vi "PlanVirtualStave.vi"(7 "Stave Locking Points [mm]":dbl[][](array[numeric])=[[0.0, 0.0, 0.0], [280.05, 0.0, 0.0], [574.05, 0.0, 0.0], [868.05, 0.0, 0.0], [1162.05, 0.0, 0.0]], 8 "Working height [mm]":dbl, 10 "Module fiducial marker":T3(ring), 11 "Tape Type":enum16{"Stereo", "Axial"}(ring)=enum."Axial") -> (0 "Module fiducials in the Stave's basis":T1(graph)=[{"Generated List of Module Coordinates"=[-7.69, 87.79, 87.79, -7.69, 90.31, 185.79000000000002, 185.79000000000002, 90.31, 188.31, 283.79, 283.79, 188.31, 286.31, 381.79, 381.79, 286.31, 384.31, 479.79, 479.79, 384.31, 482.31, 577.79, 577.79, 482.31, 580.31, 675.79, 675.79, 580.31, 678.31, 773.79, 773.79, 678.31, 776.31, 871.79, 871.79, 776.31, 874.31, 969.79, 969.79, 874.31, 972.31, 1067.79, 1067.79, 972.31, 1070.31, 1165.79, 1165.79, 1070.31, 1168.31, 1263.79, 1263.79, 1168.31], "Generated List of Module Coordinates"=[-16.132, -16.132, -113.21200000000002, -113.21200000000002, -16.132, -16.132, -113.21200000000002, -113.21200000000002, -16.132, -16.132, -113.21200000000002, -113.21200000000002, -16.132, -16.132, -113.21200000000002, -113.21200000000002, -16.132, -16.132, -113.21200000000002, -113.21200000000002, -16.132, -16.132, -113.21200000000002, -113.21200000000002, -16.132, -16.132, -113.21200000000002, -113.21200000000002, -16.132, -16.132, -113.21200000000002, -113.21200000000002, -16.132, -16.132, -113.21200000000002, -113.21200000000002, -16.132, -16.132, -113.21200000000002, -113.21200000000002, -16.132, -16.132, -113.21200000000002, -113.21200000000002, -16.132, -16.132, -113.21200000000002, -113.21200000000002, -16.132, -16.132, -113.21200000000002, -113.21200000000002]}, {"Generated List of Module Coordinates"=[0.0, 280.05, 574.05, 868.05, 1162.05], "Generated List of Module Coordinates"=[0.0, 0.0, 0.0, 0.0, 0.0]}], 3 "Generated List: Coordinates of Fiducials on Modules":dbl[][](array[numeric])=[[-7.69, -16.132, 0.0], [87.79, -16.132, 0.0], [87.79, -113.21200000000002, 0.0], [-7.69, -113.21200000000002, 0.0], [90.31, -16.132, 0.0], [185.79000000000002, -16.132, 0.0], [185.79000000000002, -113.21200000000002, 0.0], [90.31, -113.21200000000002, 0.0], [188.31, -16.132, 0.0], [283.79, -16.132, 0.0], [283.79, -113.21200000000002, 0.0], [188.31, -113.21200000000002, 0.0], [286.31, -16.132, 0.0], [381.79, -16.132, 0.0], [381.79, -113.21200000000002, 0.0], [286.31, -113.21200000000002, 0.0], [384.31, -16.132, 0.0], [479.79, -16.132, 0.0], [479.79, -113.21200000000002, 0.0], [384.31, -113.21200000000002, 0.0], [482.31, -16.132, 0.0], [577.79, -16.132, 0.0], [577.79, -113.21200000000002, 0.0], [482.31, -113.21200000000002, 0.0], [580.31, -16.132, 0.0], [675.79, -16.132, 0.0], [675.79, -113.21200000000002, 0.0], [580.31, -113.21200000000002, 0.0], [678.31, -16.132, 0.0], [773.79, -16.132, 0.0], [773.79, -113.21200000000002, 0.0], [678.31, -113.21200000000002, 0.0], [776.31, -16.132, 0.0], [871.79, -16.132, 0.0], [871.79, -113.21200000000002, 0.0], [776.31, -113.21200000000002, 0.0], [874.31, -16.132, 0.0], [969.79, -16.132, 0.0], [969.79, -113.21200000000002, 0.0], [874.31, -113.21200000000002, 0.0], [972.31, -16.132, 0.0], [1067.79, -16.132, 0.0], [1067.79, -113.21200000000002, 0.0], [972.31, -113.21200000000002, 0.0], [1070.31, -16.132, 0.0], [1165.79, -16.132, 0.0], [1165.79, -113.21200000000002, 0.0], [1070.31, -113.21200000000002, 0.0], [1168.31, -16.132, 0.0], [1263.79, -16.132, 0.0], [1263.79, -113.21200000000002, 0.0], [1168.31, -113.21200000000002, 0.0]])   [LabVIEW 2016]
panel:
  out "output cluster":cluster{dbl[], dbl[]}
  out "Y centreline":dbl
  out "Distance to EOS, x [mm]":dbl=-7.69
  in  "Module centre [mm]":T2
  in  "N modules":dbl=13.0
  out "Distance to EOS, y [mm]":dbl=-16.132
  in  "Module width [mm]":dbl=97.54
  in  "Module pitch [mm]":dbl=98.0
  # "Based on Sutcliffe Drawings:\n\nDistance to EOS, axial = [ -7.69, -16.132 ]\nstereo = [ -9.591, 115.081 ]"
  # "Provided by Camera Calibration:"
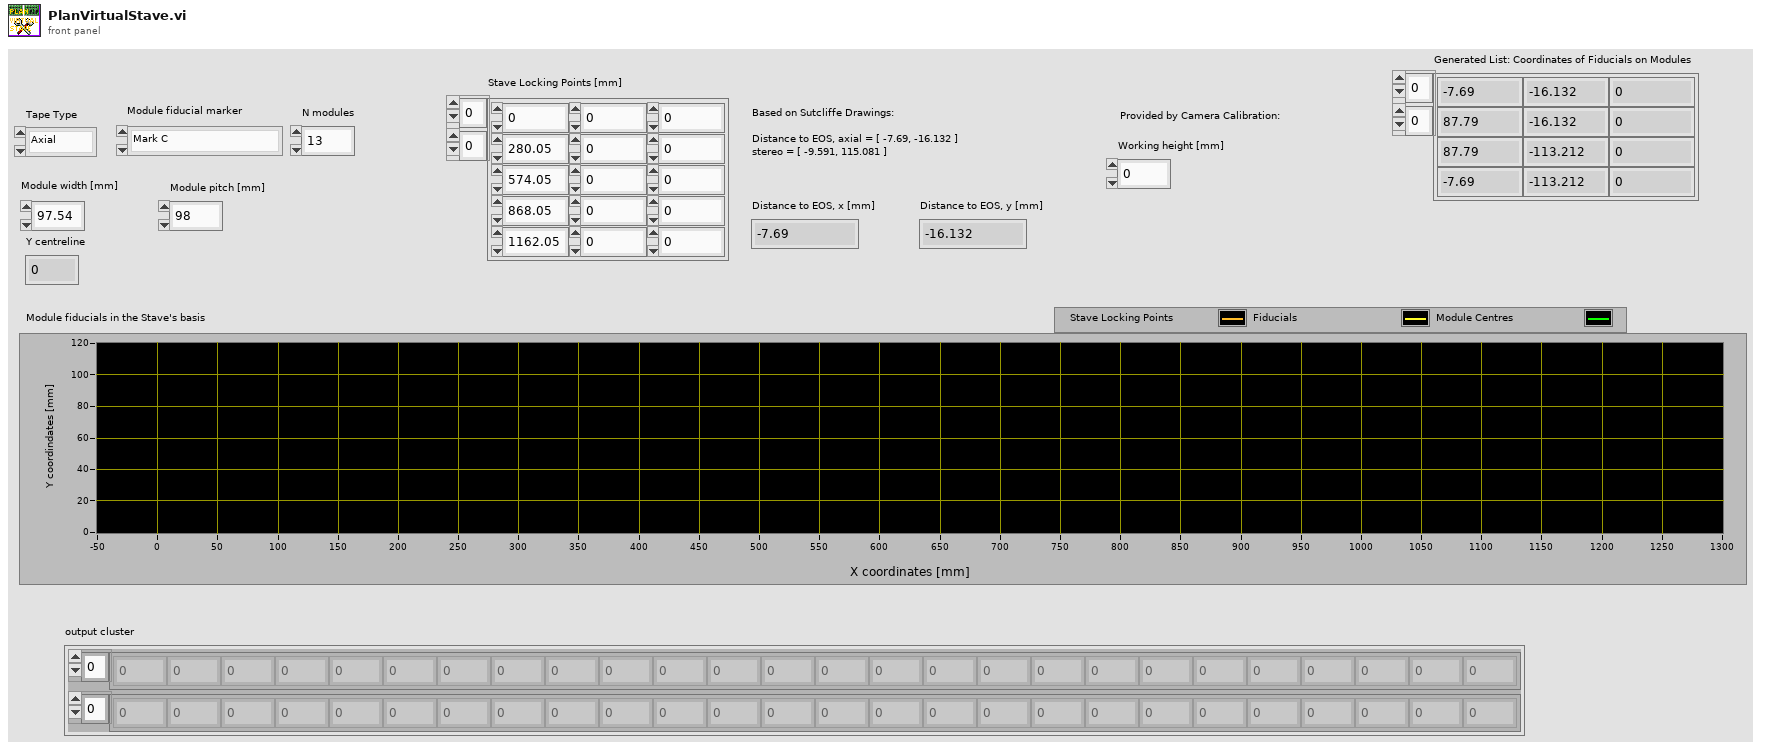
[diagram p1: front panel]
types:
  T1 = cluster{"Generated List of Module Coordinates":dbl[], "Generated List of Module Coordinates":dbl[]}[]
  T2 = cluster{"X [mm]":dbl, "Y [mm]":dbl, "Z [mm]":dbl}
  T3 = enum16{"Mark C", "Mark B", "Strip Corner", "[None]"}
  T4 = cluster{"Generated List of Module Coordinates":dbl[], "Generated List of Module Coordinates":dbl[]}
  T5 = cluster{"Stave Locking Points [mm]":dbl[], "Stave Locking Points [mm]":dbl[]}
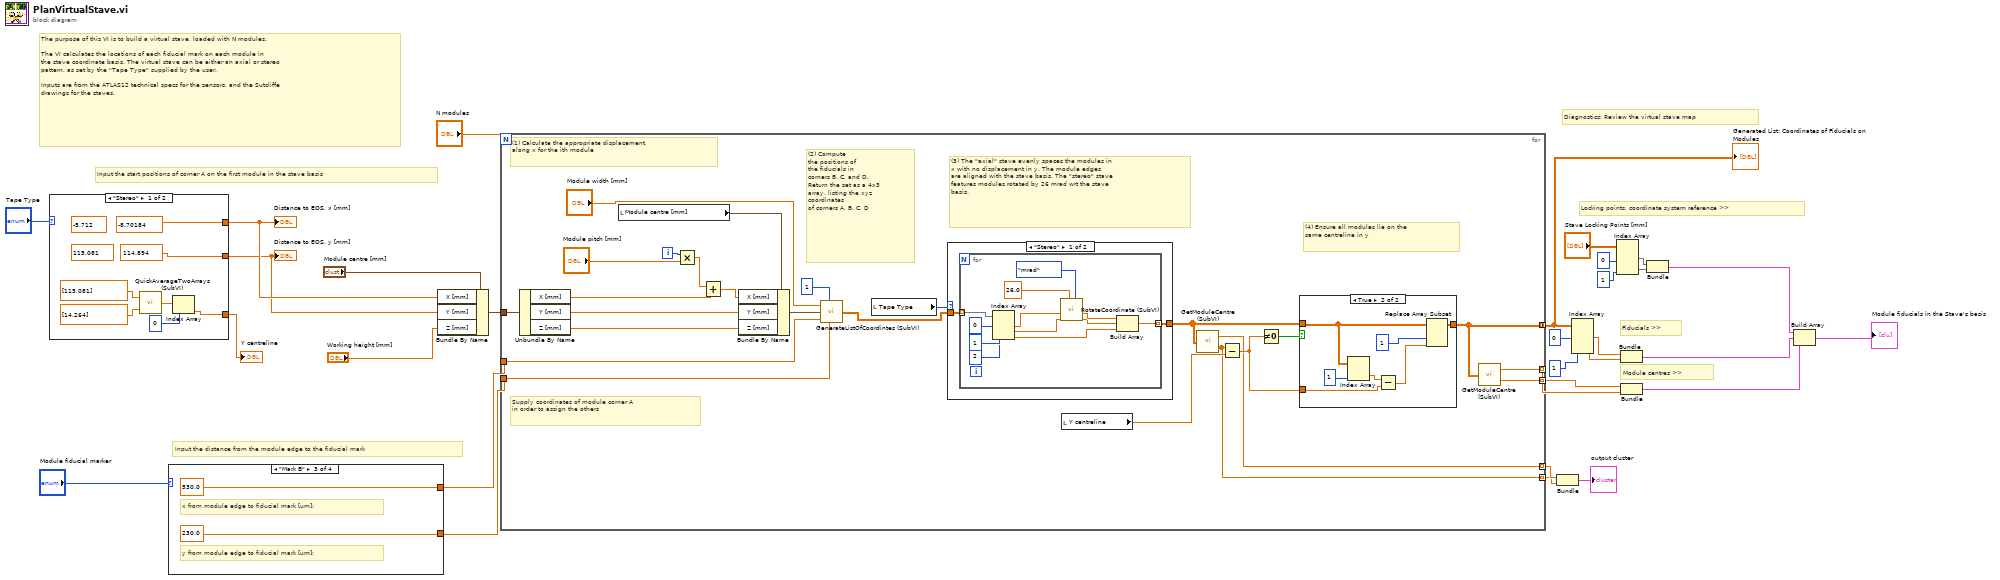
[diagram p0: block diagram]
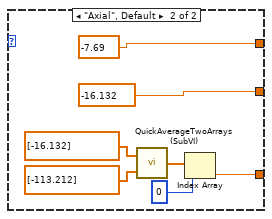
[diagram p2: hidden frame]
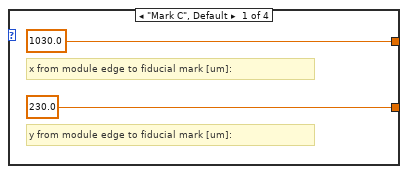
[diagram p5: hidden frame]
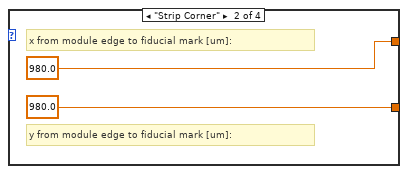
[diagram p6: hidden frame]
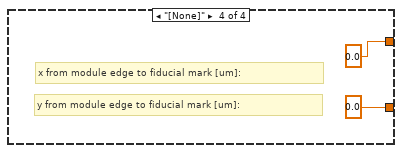
[diagram p7: hidden frame]
diagram:
  # "Locking points, coordinate system reference >>"
  # "Module centres >>"
  # "Fiducials >>"
  # "Diagnostics: Review the virtual stave map"
  # "Input the start positions of corner A on the first module in the stave basis"
  # "Input the distance from the module edge to the fiducial mark"
  # "The purpose of this VI is to build a virtual stave, loaded with N modules.\n\nThe VI calculates the locations of each fiducial mark on each module in \nthe stave coordinate basis. The virtual stave can be either an axial or stereo \npattern, as set by the \"Tape Type\" supplied by the user.\n\nInputs are from the ATLAS12 technical specs for the sensors, and the Sutcliffe\ndrawings for the staves."
  n1 = case shown="\"Stereo\"" "Tape Type" {
    tunnel: [-8.70184 -7.69] -> w15
    tunnel: [114.894 -16.132] -> w14
    tunnel: [w31 w38] -> w4
    frame "Stereo" {
      (unwired) 115.081
      (unwired) -5.712
      n2 = call "QuickAverageTwoArrays (SubVI).vi"("B"=dbl[] [14.264], "A"=dbl[] [115.081]) -> ("Average of A and B"=w33:dbl[])
      n3 = Index Array(array=w33, index=0) -> (element=w31:dbl)
    }
    frame "Axial", Default {
      n4 = call "QuickAverageTwoArrays (SubVI).vi"("B"=dbl[] [-113.212], "A"=dbl[] [-16.132]) -> ("Average of A and B"=w40:dbl[])
      n5 = Index Array(array=w40, index=0) -> (element=w38:dbl)
    }
  }
  "Distance to EOS, y [mm]" <- w14
  "Distance to EOS, x [mm]" <- w15
  "Y centreline" <- w4
  n6 = case shown="\"Mark B\"" "Module fiducial marker" {
    tunnel: [1030.0 980.0 530.0 0.0] -> w29
    tunnel: [230.0 980.0 230.0 0.0] -> w28
    frame "Mark C", Default {
      # "y from module edge to fiducial mark [um]:"
      # "x from module edge to fiducial mark [um]:"
    }
    frame "Strip Corner" {
      # "y from module edge to fiducial mark [um]:"
      # "x from module edge to fiducial mark [um]:"
    }
    frame "Mark B" {
      # "y from module edge to fiducial mark [um]:"
      # "x from module edge to fiducial mark [um]:"
    }
    frame "[None]" {
      # "y from module edge to fiducial mark [um]:"
      # "x from module edge to fiducial mark [um]:"
    }
  }
  n7 = Bundle By Name(cluster="Module centre [mm]", "X [mm]"=w15, "Y [mm]"=w14, "Z [mm]"="Working height [mm]") -> (w22:T2)
  n8 = for {
    N: "N modules" -> [_]
    tunnel: w29 -> [w66]
    tunnel: w28 -> [w76]
    tunnel: w22 -> [w65]
    tunnel: [w58] -> w13 mode=concatenating
    tunnel: [w57] -> w10 mode=indexing
    tunnel: [w56] -> w9 mode=indexing
    tunnel: [w54] -> w3 mode=indexing
    tunnel: [w53] -> w2 mode=indexing
    i -> [w75]
    # "(4) Ensure all modules lie on the \nsame centreline in y"
    # "(3) The \"axial\" stave evenly spaces the modules in \nx with no displacement in y. The module edges \nare aligned with the stave basis. The \"stereo\" stave \nfeatures modules rotated by 26 mrad wrt the stave\nbasis."
    # "(2) Compute\nthe positions of \nthe fiducials in \ncorners B, C, and D. \nReturn the set as a 4x3\narray, listing the xyz \ncoordinates\nof corners A, B, C, D"
    # "(1) Calculate the appropriate displacement \nalong x for the ith module"
    # "Supply coordinates of module corner A \nin order to assign the others"
    n9 = Unbundle By Name(w65) -> ("X [mm]"=w74:dbl, "Y [mm]"=w72:dbl, "Z [mm]"=w70:dbl)
    n10 = local read "Module centre [mm]"() -> (w68:T2)
    n11 = Multiply(x=w75, y="Module pitch [mm]") -> (x*y=w73:dbl)
    n12 = Add(x=w73, y=w74) -> (x+y=w71:dbl)
    n13 = Bundle By Name(cluster=w68, "X [mm]"=w71, "Y [mm]"=w72, "Z [mm]"=w70) -> (w69:T2)
    n14 = call "GenerateListOfCoordintes (SubVI).vi"("Module side length [mm]"="Module width [mm]", "Nloops"=1, "A [mm]"=w69, "x to fiducial [um]"=w66, "y to fiducial [um]"=w76) -> ("Generated List of Module Coordinates"=w62:dbl[][])  [unwired: 4 in]
    n15 = local read "Tape Type"() -> (w64:enum16{"Stereo", "Axial"})
    n16 = case shown="\"Stereo\"" w64 {
      tunnel: [w87 w100] -> w60
      tunnel: w62 -> [w86 w100]
      frame "Stereo" {
        n17 = for {
          tunnel: [w89] -> w87 mode=indexing
          tunnel: w86 -> [w88] mode=indexing
          n18 = Index Array(array=w88, index #1=0 ("index"), index #2=1 ("index"), index #3=2 ("index")) -> (element #1=w94:dbl, element #2=w93:dbl, element #3=w90:dbl)
          n19 = call "RotateCoordinate (SubVI).vi"("Units"=enum16{"mrad", "Radians", "Degrees"}."mrad", "Angle"=26.0, "y"=w93, "x"=w94) -> ("y'"=w91:dbl, "x'"=w92:dbl)  [unwired: 6 in]
          n20 = Build Array(w92, w91, w90) -> (w89:dbl[])
        }
      }
      frame "Axial", Default {
      }
    }
    n21 = local read "Y centreline"() -> (w63:dbl)
    n22 = call "GetModuleCentre (SubVI).vi"("4x3 Array of Fiducial Coordinates"=w60) -> ("x, centre"=w54:dbl, "y, centre"=w53:dbl)
    n23 = Subtract(x=w53, y=w63) -> (x-y=w59:dbl)
    n24 = Not Equal To 0?(x=w59) -> (x != 0?=w61:bool)
    n25 = case shown="True" w61 {
      tunnel: w60 -> [w78 w85]
      tunnel: w59 -> [_ w80]
      tunnel: [w78 w79] -> w58
      frame False {
      }
      frame True {
        n26 = Index Array(array=w85, index (col)=1 ("disabled index (col)")) -> (element=w83:dbl[])  [unwired: 1 in]
        n27 = Subtract(x=w83, y=w80) -> (x-y=w82:dbl[])
        n28 = Replace Array Subset(array=w85, new element=w82, index (col)=1 ("disabled index (col)")) -> (w79:dbl[][])  [unwired: 1 in]
      }
    }
    n29 = call "GetModuleCentre (SubVI).vi"("4x3 Array of Fiducial Coordinates"=w58) -> ("x, centre"=w57:dbl, "y, centre"=w56:dbl)
  }
  "Generated List: Coordinates of Fiducials on Modules" <- w13
  n30 = Bundle(w3, w2) -> (→"output cluster":cluster{dbl[], dbl[]})  [unwired: 1 in]
  n31 = Index Array(array=w13, index (col) #1=0 ("disabled index (col)"), index (col) #2=1 ("index (col)")) -> (element #1=w27:dbl[], element #2=w26:dbl[])  [unwired: 2 in]
  n32 = Index Array(array="Stave Locking Points [mm]", index (col) #1=0 ("disabled index (col)"), index (col) #2=1 ("disabled index (col)")) -> (element #1=w18:dbl[], element #2=w17:dbl[])  [unwired: 2 in]
  n33 = Bundle("Generated List of Module Coordinates"=w27, "Generated List of Module Coordinates"=w26) -> (w8:T4)  [unwired: 1 in]
  n34 = Bundle(w10, w9) -> (w7:cluster{dbl[], dbl[]})  [unwired: 1 in]
  n35 = Bundle("Stave Locking Points [mm]"=w18, "Stave Locking Points [mm]"=w17) -> (w6:T5)  [unwired: 1 in]
  n36 = Build Array(w6, w8, w7) -> (→"Module fiducials in the Stave's basis":T1)
